vi "DAQ.Get Device from Channel Name.vi"(11 "Channel":tag) -> (3 "Device":tag)   [LabVIEW 2019, in "Instrument.Lockin.lvlib" / "Instrument.DAQ.lvclass"]
uses:
  Instrument.DAQ.lvclass
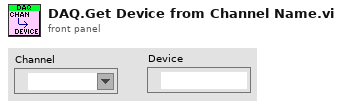
[diagram p1: front panel]
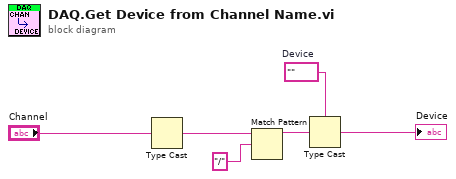
[diagram p0: block diagram]
diagram:
  w5 = tag ""  # Device
  n1 = Type Cast(x="Channel") -> (*(type *) &x=w1:string)  [unwired: 1 in]
  n2 = Match Pattern(string=w1, regular expression="/") -> (before substring=w4:string)  [unwired: 1 in, 3 out]
  n3 = Type Cast(type=w5, x=w4) -> (*(type *) &x=→"Device":tag)
